vi "Finding HB Center.vi"() -> ()   [LabVIEW 2021, in "Test VIs.lvclass"]
uses:
  Test VIs/Test VIs.lvclass
  Classes/Workspace/Workspace.ctl
  Classes/Workspace/Component/Component Tray.lvclass
  Classes/Controller/Controller.lvclass
  Classes/Workspace/Fixture.lvclass
panel:
  out "error out":errorcluster
  in  "error in (no error)":errorcluster
  out "Workspace":T1
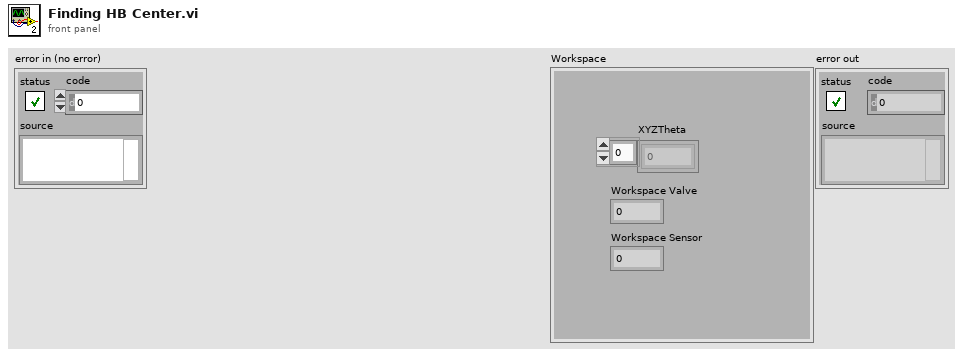
[diagram p1: front panel]
types:
  T1 = typedef "Fixture.lvclass/Workspace.ctl" = cluster{"XYZTheta":dbl[], "Workspace Valve":i32, "Workspace Sensor":i32}
  T2 = typedef "Controller.lvclass/Controllers.ctl" = cluster{"I-O.lvclass":refnum<class "I-O.lvclass">, "Gantry":refnum<k24>, "Dispenser":refnum<visa-resource-name>}
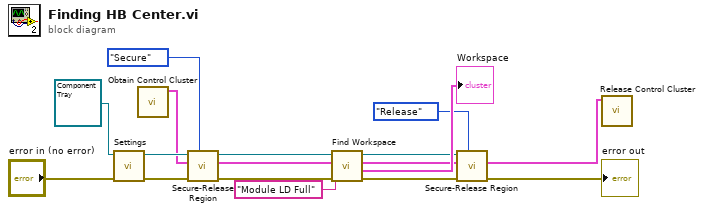
[diagram p0: block diagram]
diagram:
  n1 = call-dynamic "Settings.vi"("error in (no error)"="error in (no error)", "Component in"=refnum<class "Component Tray.lvclass"> refnum ("Component Tray.lvclass")) -> ("error out"=w5:errorcluster, "Component out"=w15:refnum<class "Component Tray.lvclass">)  [unwired: 8 in]
  n2 = call "Obtain Control Cluster.vi"() -> ("Control Out"=w12:T2)  [unwired: 10 in, 1 out]
  n3 = call-dynamic "Secure-Release Region.vi"("Action"=enum16{"Secure", "Release"}."Secure", "error in (no error)"=w5, "Control In"=w12, "Workspace in"=w15) -> ("error out"=w4:errorcluster, "Control Out"=w11:T2, "Workspace out"=w10:refnum<class "Component Tray.lvclass">)  [unwired: 4 in, 1 out]
  n4 = call-dynamic "Find Workspace.vi"("error in (no error)"=w4, "Assembly Type"="Module LD Full", "Control In"=w11, "Component.lvclass"=w10) -> ("error out"=w3:errorcluster, "Workspace"=→"Workspace":T1, "Control Out"=w8:T2, "Workspace Out"=w9:refnum<class "Component Tray.lvclass">)  [unwired: 4 in]
  n5 = call-dynamic "Secure-Release Region.vi"("Action"=enum16{"Secure", "Release"}."Release", "error in (no error)"=w3, "Control In"=w8, "Workspace in"=w9) -> ("error out"=→"error out":errorcluster, "Control Out"=w7:T2)  [unwired: 4 in, 2 out]
  n6 = call "Release Control Cluster.vi"("output cluster"=w7) -> ()  [unwired: 11 in]
